vi "gaussianGuesses.vi"(10 "X Values":dbl[](array[numeric]), 11 "Y Values":dbl[](array[numeric])) -> (2 "Guesses":dbl[](array[numeric]) caption="Initial Gaussian Fit Guesses", 3 "FWHMScaling":dbl)   [LabVIEW 2011]
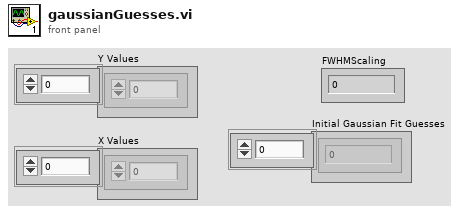
[diagram p1: front panel]
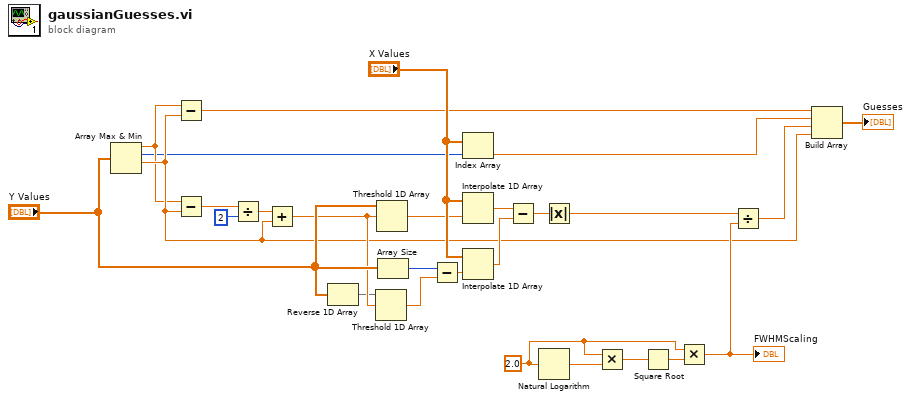
[diagram p0: block diagram]
diagram:
  w4 = 2.0
  n1 = Array Max & Min(array="Y Values") -> (max value=w8:dbl, max index (indices)=w5:i32, min value=w12:dbl)  [unwired: 1 out]
  n2 = Subtract(x=w8, y=w12) -> (x-y=w7:dbl)
  n3 = Subtract(x=w8, y=w12) -> (x-y=w9:dbl)
  n4 = Divide(x=w9, y=2) -> (x/y=w11:dbl)
  n5 = Add(x=w11, y=w12) -> (x+y=w14:dbl)
  n6 = Reverse 1D Array(array="Y Values") -> (reversed array=w13:dbl[])
  n7 = Threshold 1D Array(2:w14, 3:w13) -> (0:w16:dbl)  [unwired: 1 in]
  n8 = Threshold 1D Array(2:w14, 3:"Y Values") -> (0:w15:dbl)  [unwired: 1 in]
  n9 = Array Size(array="Y Values") -> (size(s)=w17:i32)
  n10 = Subtract(x=w17, y=w16) -> (x-y=w18:dbl)
  n11 = Index Array(array="X Values", index=w5) -> (element=w6:dbl)
  n12 = Interpolate 1D Array(1:w15, 2:"X Values") -> (0:w19:dbl)
  n13 = Interpolate 1D Array(1:w18, 2:"X Values") -> (0:w20:dbl)
  n14 = Subtract(x=w19, y=w20) -> (x-y=w21:dbl)
  n15 = Natural Logarithm(1:w4) -> (0:w1:dbl)
  n16 = Absolute Value(x=w21) -> (abs(x)=w22:dbl)
  n17 = Multiply(x=w4, y=w1) -> (x*y=w2:dbl)
  n18 = Square Root(x=w2) -> (sqrt(x)=w3:dbl)
  n19 = Multiply(x=w4, y=w3) -> (x*y=w27:dbl)
  "FWHMScaling" <- w27
  n20 = Divide(x=w22, y=w27) -> (x/y=w23:dbl)
  n21 = Build Array(w7, w6, w23, w12) -> (→"Guesses":dbl[])
